vi "PXI6704_ao.vi"() -> ()   [LabVIEW 2017]
doc: "Use this template to build a producer/consumer design pattern with events to produce queue items. Use this design pattern instead of the User Interface Event Handler pattern for user interfaces when you want to execute code asynchronously in response to an event without slowing the user interface responsiveness."
panel:
  in  "Run":bool
  in  "All Current":bool
  in  "电流":i32(listbox)
  in  "All Volt":bool
  in  "电压":i32(listbox)
  in  "Enqueue Element":bool
  in  "stop":bool
  # "PXI-6704模拟信号发生器"
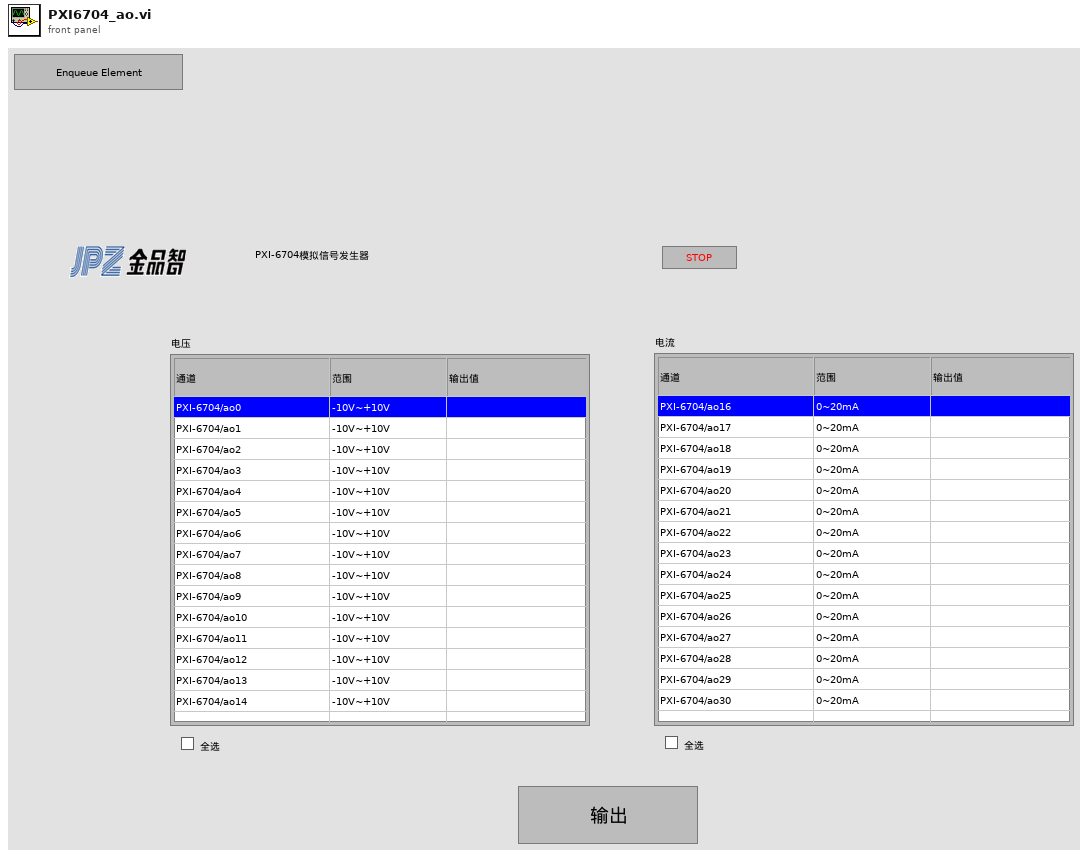
[diagram p1: front panel]
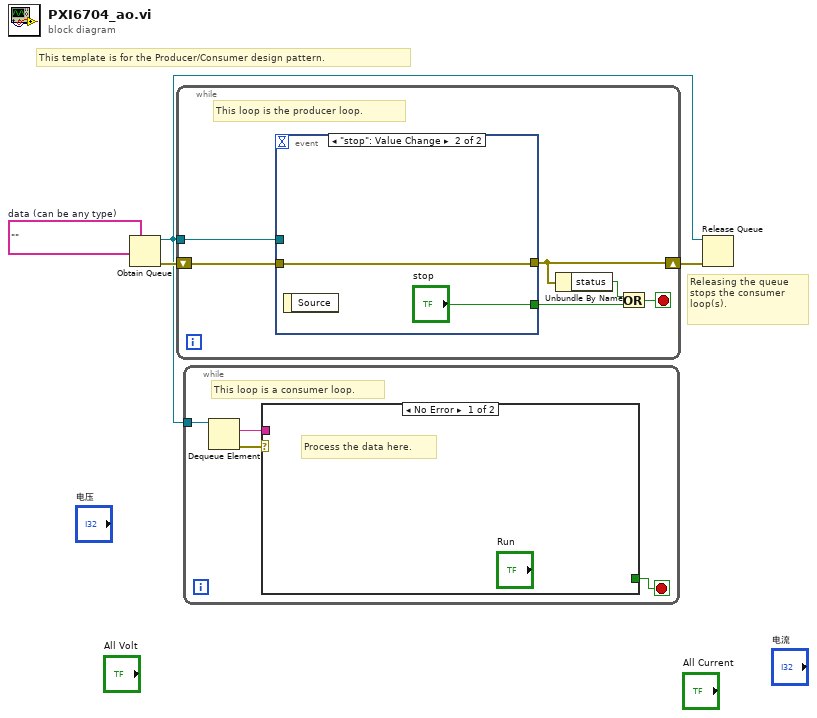
[diagram p0: block diagram]
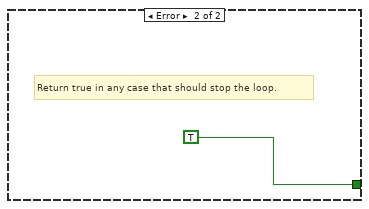
[diagram p2: hidden frame]
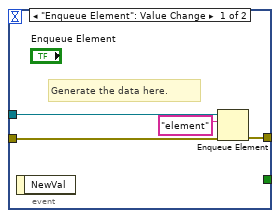
[diagram p3: hidden frame]
diagram:
  w2 = ""  # data (can be any type)
  # "Releasing the queue stops the consumer loop(s)."
  # "This template is for the Producer/Consumer design pattern."
  n1 = Obtain Queue(element data type=w2) -> (queue out=w1:refnum<queue>, error out=w4:errorcluster)  [unwired: 4 in, 1 out]
  n2 = while {
    shift-right: [w6] -> w3
    shift-left: w4 -> [w9]
    tunnel: w1 -> [w10]
    stop <- w7 stop-if-true
    # "This loop is the producer loop."
    n3 = event shown="[1] \"stop\": Value Change" {
      selector: _ -> [_ _]
      dyn-events: _ -> [_ _]
      timeout: _ -> [_ _]
      tunnel: w10 -> [w14 _]
      tunnel: w9 -> [w13 w15]
      tunnel: [w12 w15] -> w6
      tunnel: [_ "stop"] -> w8
      event "Enqueue Element": Value Change {
        # "Generate the data here."
        n4 = event-data() -> ()  [unwired: 1 in, 1 out]
        n5 = Enqueue Element(queue=w14, element="element", error in (no error)=w13) -> (error out=w12:errorcluster)  [unwired: 1 in, 2 out]
      }
      event "stop": Value Change {
        n6 = event-data() -> ()  [unwired: 1 in, 1 out]
      }
    }
    n7 = Unbundle By Name(w6) -> ("status"=w5:bool)
    n8 = Or(x=w5, y=w8) -> (x .or. y?=w7:bool)
  }
  n9 = while {
    tunnel: w1 -> [w20]
    stop <- w17 stop-if-true
    # "This loop is a consumer loop."
    n10 = Dequeue Element(queue=w20) -> (element=w18:string, error out=w19:errorcluster)  [unwired: 2 in, 2 out]
    n11 = case shown="No Error" w19 {
      tunnel: w18 -> [_ _]
      tunnel: [_ TRUE] -> w17
      frame No Error {
        # "Process the data here."
      }
      frame Error {
        # "Return true in any case that should stop the loop."
      }
    }
  }
  n12 = Release Queue(queue=w1, error in (no error)=w3) -> ()  [unwired: 1 in, 3 out]
